vi "Read Multi Eval Meas PVT Trace Results.vi"(8 "error in (no error)":errorcluster, 9 "Result Type (Current)":i32(ring) items=["Current"=0, "Average"=1, "Maximum"=4, "Minimum"=5], 10 "Instance (1)":i32=1, 11 "VISA resource name":refnum<visa-resource-name>) -> (0 "error out":errorcluster, 1 "Results":dbl[](array[numeric]) format="%^.3e", 2 "Reliability":i32, 3 "VISA resource name out":refnum<visa-resource-name>)   [LabVIEW 2015, in "Rohde&Schwarz CMP LR WPAN Measurement.lvlib"]
doc: "Starts a new single shot measurement and returns the power vs time traces. Eight values per chip are returned, starting from 500-st chip before the first chip to 500-st chip after the last chip in the burst.\n\nAttribute:\n-\n\nRemote-control commands:\nREAD:WPAN:MEAS<i>:MEValuation:TRACe:PVTime:CURRent?\nREAD:WPAN:MEAS<i>:MEValuation:TRACe:PVTime:AVERage?\nREAD:WPAN:MEAS<i>:MEValuation:TRACe:PVTime:MAXimum?\nREAD:WPAN:MEAS<i>:MEValuation:TRACe:PVTime:MINimum?"
uses:
  <instrlib>/Rohde&Schwarz CMP LR WPAN Measurement/Rohde&Schwarz CMP LR WPAN Measurement.lvlib
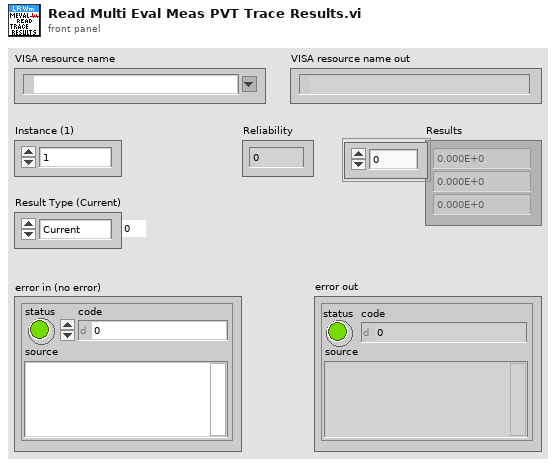
[diagram p1: front panel]
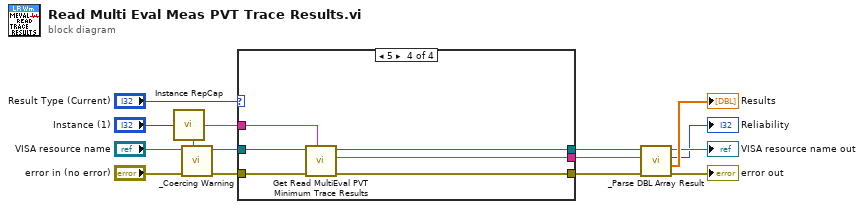
[diagram p0: block diagram]
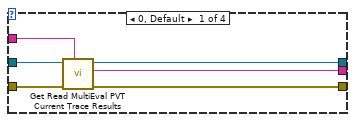
[diagram p2: hidden frame]
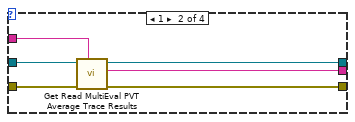
[diagram p3: hidden frame]
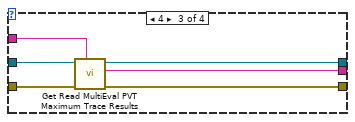
[diagram p4: hidden frame]
diagram:
  n1 = call <instrlib>:"Instance RepCap.vi"("Instance In"="Instance (1)") -> ("In Range?"=w14:bool, "RepCap Identifier Out"=w15:string)  [unwired: 1 in]
  n2 = call <instrlib>:"_Coercing Warning.vi"("In Range?"=w14, "error in (no error)"="error in (no error)", "VISA resource name"="VISA resource name") -> ("error out"=w10:errorcluster, "VISA resource name out"=w9:refnum<visa-resource-name>)  [unwired: 7 in]
  n3 = case shown="5" "Result Type (Current)" {
    tunnel: w15 -> [w21 w27 w31 w39]
    tunnel: w9 -> [w20 w26 w32 w37]
    tunnel: w10 -> [w19 w25 w33 w38]
    tunnel: [w16 w22 w28 w34] -> w5
    tunnel: [w18 w24 w30 w36] -> w4
    tunnel: [w17 w23 w29 w35] -> w3
    frame 0, Default {
      n4 = call "Get Read MultiEval PVT Current Trace Results"("Repeated Capabilities"=w21, "error in (no error)"=w19, "instrument handle"=w20) -> ("error out"=w16:errorcluster, "Read MultiEval PVT Current Trace Results"=w17:string, "instrument handle out"=w18:refnum<visa-resource-name>)  [unwired: 6 in]
    }
    frame 1 {
      n5 = call "Get Read MultiEval PVT Average Trace Results"("Repeated Capabilities"=w27, "error in (no error)"=w25, "instrument handle"=w26) -> ("error out"=w22:errorcluster, "Read MultiEval PVT Average Trace Results"=w23:string, "instrument handle out"=w24:refnum<visa-resource-name>)  [unwired: 6 in]
    }
    frame 4 {
      n6 = call "Get Read MultiEval PVT Maximum Trace Results"("Repeated Capabilities"=w31, "error in (no error)"=w33, "instrument handle"=w32) -> ("error out"=w28:errorcluster, "Read MultiEval PVT Maximum Trace Results"=w29:string, "instrument handle out"=w30:refnum<visa-resource-name>)  [unwired: 6 in]
    }
    frame 5 {
      n7 = call "Get Read MultiEval PVT Minimum Trace Results"("Repeated Capabilities"=w39, "error in (no error)"=w38, "instrument handle"=w37) -> ("error out"=w34:errorcluster, "Read MultiEval PVT Minimum Trace Results"=w35:string, "instrument handle out"=w36:refnum<visa-resource-name>)  [unwired: 6 in]
    }
  }
  n8 = call <instrlib>:"_Parse DBL Array Result.vi"("error in (no error)"=w5, "Input String"=w3, "VISA resource name"=w4) -> ("error out"=→"error out":errorcluster, "Results"=→"Results":dbl[], "Reliability"=→"Reliability":i32, "VISA resource name out"=→"VISA resource name out":refnum<visa-resource-name>)  [unwired: 5 in]
